vi "App_Simulator Data(FGV).vi"(6 "Simulator Data Method(Get)":T1, 8 "error in":errorcluster) -> (0 "error out":errorcluster, 3 "Data":waveform(dbl))   [LabVIEW 2015, in "Application 2.lvlib"]
uses:
  Application 2.lvlib
  Data Def/App_Simulator Data Method.ctl
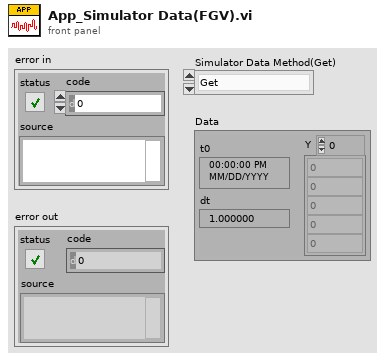
[diagram p1: front panel]
types:
  T1 = typedef "Application 2.lvlib/App_Simulator Data Method.ctl" = enum16{"Get", "Put"}
  T2 = enum16{"Get Normal Standard Sample", "Get Hypokalemia Standard Sample", "Get Ventricular Tachycardia Standard Sample", "Get Hyperkalemia Standard Sample", "Get Testing Sample"}
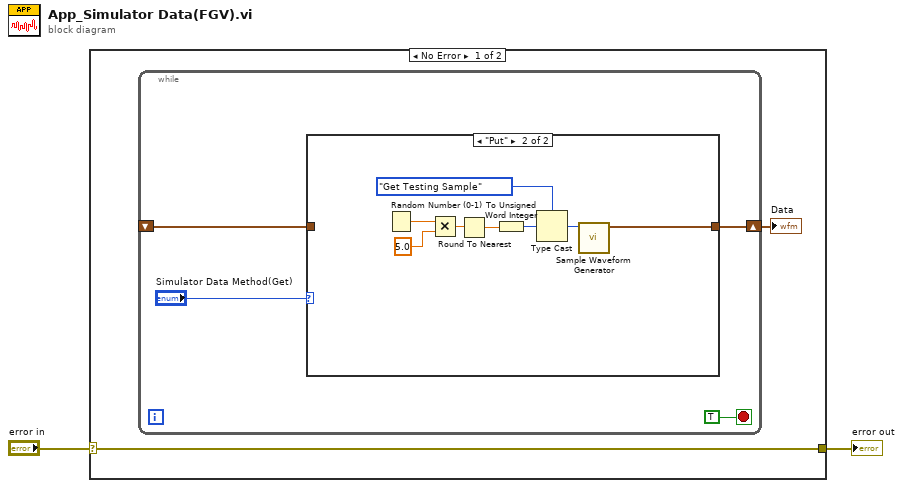
[diagram p0: block diagram]
diagram:
  n1 = case shown="No Error" "error in" {
    selector: "error in" -> [w3 w18]
    tunnel: [w3 w18] -> w1
    frame No Error {
      n2 = while {
        shift-right: [w6] -> w4
        shift-left: _ -> [w5]
        stop <- TRUE stop-if-true
        n3 = case shown="\"Put\"" "Simulator Data Method(Get)" {
          tunnel: [w9 w10] -> w6
          tunnel: w5 -> [w9 _]
          frame "Get", Default {
          }
          frame "Put" {
            n4 = Random Number (0-1)() -> (number: 0 to 1=w17:dbl)
            n5 = Multiply(x=w17, y=5.0) -> (x*y=w15:dbl)
            n6 = Round To Nearest(number=w15) -> (nearest integer value=w14:dbl)
            n7 = To Unsigned Word Integer(number=w14) -> (unsigned 16bit integer=w13:u16)
            n8 = Type Cast(type=T2."Get Testing Sample" ("Action"), x=w13) -> (*(type *) &x=w11:T2)
            n9 = call "Sample Waveform Generator.vi"("Action"=w11) -> ("Sample Waveform"=w10:waveform(dbl))  [unwired: 10 in]
          }
        }
      }
      "Data" <- w4
    }
    frame Error {
    }
  }
  "error out" <- w1
